vi "LMSmy.vi"(8 "sample length":i32=100, 9 "x(n+1) input point":dbl format="%0.2f", 10 "error e(n)":dbl, 11 "mu":dbl) -> (1 "y(n+1)":dbl format="%.2f", 2 "w(n)":dbl[](array[numeric]))   [LabVIEW 2020]
uses:
  <vilib>/Analysis/baseanly.llb/Real Dot Product.vi
  <vilib>/ptbypt/NI_PtbyPt.lvlib
  <vilib>/Analysis/NI_AALBase.lvlib
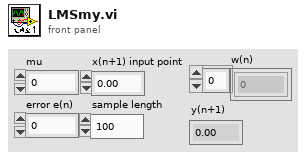
[diagram p1: front panel]
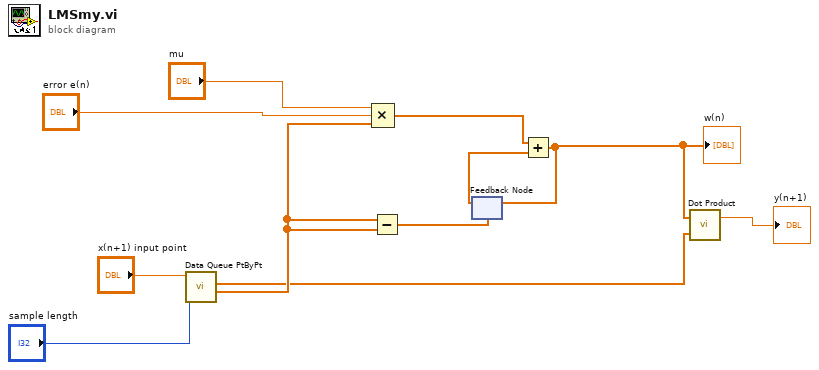
[diagram p0: block diagram]
diagram:
  n1 = call <vilib>:"Data Queue PtByPt.vi"("sample length"="sample length", "input data point"="x(n+1) input point") -> ("Previous Queue"=w7:dbl[], "Current Queue"=w3:dbl[])  [unwired: 5 in, 3 out]
  n2 = Compound Arithmetic op=MULTIPLY("mu", "error e(n)", w7) -> (w11:dbl[])
  n3 = Subtract(x=w7, y=w7) -> (x-y=w4:dbl[])
  n4 = feedback #1(w4) -> (w10:dbl[])
  n5 = Add(x=w11, y=w10) -> (x+y=w6:dbl[])
  "w(n)" <- w6
  n6 = feedback-in #1(w6) -> ()
  n7 = call-poly <vilib>:"Dot Product.vi"("Y Vector"=w3, "X Vector"=w6) -> ("X * Y"=→"y(n+1)":dbl)  [unwired: 1 out]
